vi "Update Method Result.vi"(9 "Status":T1=enum."Passed", 10 "Case":string, 11 "Test Tree In":refnum<class "Test Result Tree V2.lvclass">) -> (3 "Test Tree Out":refnum<class "Test Result Tree V2.lvclass">)   [LabVIEW 2020, in "Test Result Tree V2.lvclass"]
uses:
  Test Result Tree V2.lvclass
  C:/Git/astemes-lunit/source/Rewrite Project/Test Tree/Test Tree.lvclass
  Result/Status.ctl
  Test Tree/Test Tree.lvclass/Test Tree.ctl
  Test Tree/Test Tree.lvclass
  Utilities/LUnit Utilities.lvlib
  Result/Result.lvlib
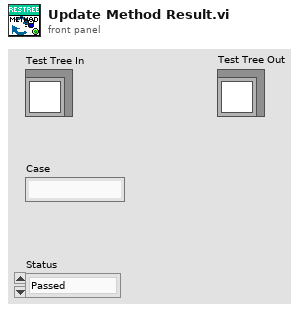
[diagram p1: front panel]
types:
  T1 = typedef "Result.lvlib/Status.ctl" = enum16{"", "Passed", "Failed", "Error", "Skipped", "Setup Error", "Broken", "Teardown Error"}
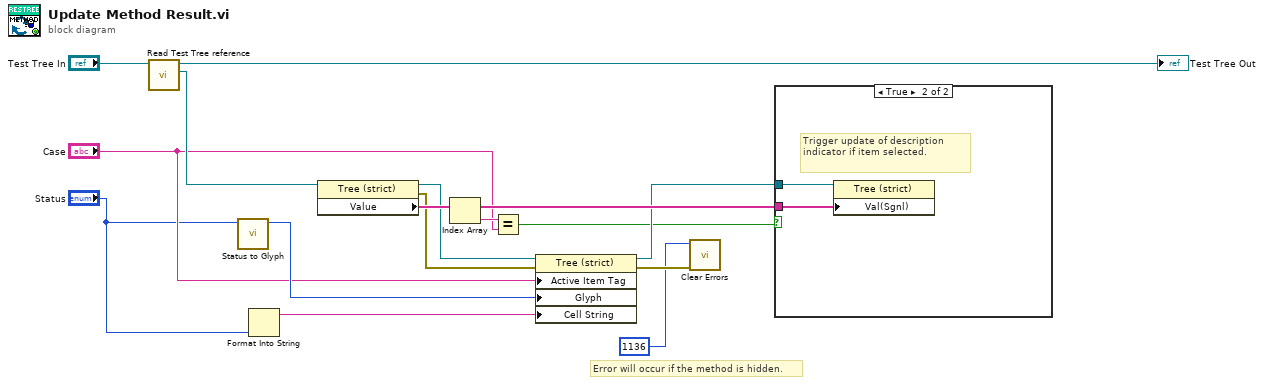
[diagram p0: block diagram]
diagram:
  # "Error will occur if the method is hidden."
  n1 = call "Read Test Tree reference.vi"("Test Tree in"="Test Tree In") -> ("Test Tree reference"=w4:refnum<vi>, "Test Tree out"=→"Test Tree Out":refnum<class "Test Result Tree V2.lvclass">)  [unwired: 8 in, 1 out]
  n2 = call "Status to Glyph.vi"("Status"="Status") -> ("Listbox Symbol Ring Constant"=w3:i32)  [unwired: 10 in]
  n3 = Format Into String("Status") -> (resulting string=w15:string)  [unwired: 3 in, 1 out]
  n4 = property on="Property Node" class="Tree (strict)"(reference=w4) -> (reference out=w9:refnum<vi>, error out=w10:errorcluster, "Value"=w13:string[])  [unwired: 1 in]
  n5 = Index Array(array=w13) -> (element=w14:string)  [unwired: 1 in]
  n6 = Equal?(x=w14, y="Case") -> (x = y?=w8:bool)
  n7 = property class="Tree (strict)"(reference=w9, error in=w10, "Active Item Tag"="Case", "Glyph"=w3, "Cell String"=w15) -> (reference out=w12:refnum<vi>, error out=w11:errorcluster)
  n8 = call <vilib>:"Clear Errors.vi"("error in (no error)"=w11, "specific error code to clear (0: all)"=1136) -> ()  [unwired: 4 in, 2 out]
  n9 = case shown="True" w8 {
    tunnel: w13 -> [_ w17]
    tunnel: w12 -> [_ w16]
    frame False {
    }
    frame True {
      # "Trigger update of description indicator if item selected."
      n10 = property on="Property Node" class="Tree (strict)"(reference=w16, "Val(Sgnl)"=w17) -> ()  [unwired: 1 in, 2 out]
    }
  }
